vi "passIfReentrant.vi"(8 "error in (no error)":errorcluster, 9 "required setting (reentrant)":T1, 10 "VI Refnum":refnum<vi>, 11 "TestCase in":refnum<class "TestCase.lvclass">) -> (0 "error out":errorcluster, 3 "TestCase out":refnum<class "TestCase.lvclass">)   [LabVIEW 2013, in "EasyXML_XML_Subset_Evaluations.lvclass"]
doc: "Tests whether the VI specified by <b>VI Refnum</b> is reentrant or non-reentrant, as specified by <b>required setting</b>"
uses:
  EasyXML_XML_Subset_Evaluations.lvclass
  <vilib>/addons/_JKI Toolkits/VI Tester/TestCase.llb/TestCase.lvclass
  EasyXMLTest/Test Support/Reentrant Setting Requirement - Enum.ctl
  EasyXMLTest/EasyXMLTest.lvclass
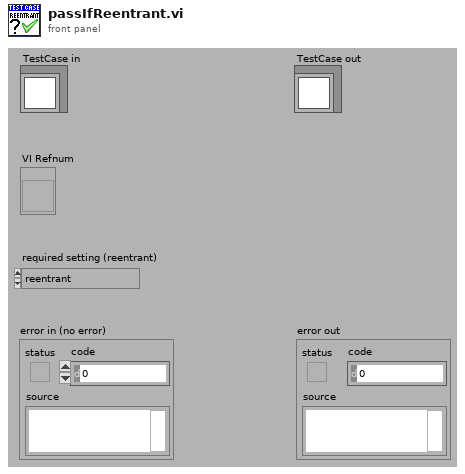
[diagram p1: front panel]
types:
  T1 = typedef "EasyXMLTest.lvclass/Reentrant Setting Requirement - Enum.ctl" = enum16{"reentrant", "non-reentrant"}
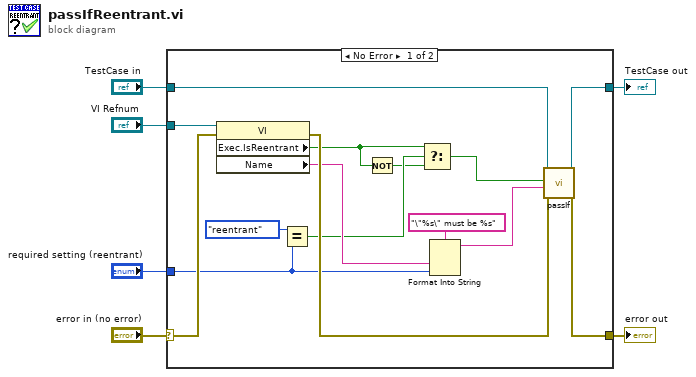
[diagram p0: block diagram]
diagram:
  n1 = case shown="No Error" "error in (no error)" {
    selector: "error in (no error)" -> [w13 w23]
    tunnel: [w19 w23] -> w5
    tunnel: [w18 w22] -> w4
    tunnel: "TestCase in" -> [w17 w22]
    tunnel: "VI Refnum" -> [w14 _]
    tunnel: "required setting (reentrant)" -> [w11 _]
    frame No Error {
      n2 = property class="VI"(reference=w14, error in=w13) -> (error out=w21:errorcluster, "Exec.IsReentrant"=w8:bool, "Name"=w15:string)  [unwired: 1 out]
      n3 = Equal?(x=Reentrant_Setting_Requirement_-_Enum."reentrant" ("required setting (reentrant)"), y=w11) -> (x = y?=w10:bool)
      n4 = Not(x=w8) -> (.not. x?=w7:bool)
      n5 = Select(t=w8, s=w10, f=w7) -> (s? t:f=w9:bool)
      n6 = Format Into String(format string="\"%s\" must be %s", w15, w11) -> (resulting string=w20:string)  [unwired: 2 in, 1 out]
      n7 = call-dynamic "passIf.vi"("error in (no error)"=w21, "message (\"\")"=w20, "pass"=w9, "TestCase in"=w17) -> ("error out"=w19:errorcluster, "TestCase out"=w18:refnum<class "TestCase.lvclass">)  [unwired: 6 in]
    }
    frame Error {
    }
  }
  "error out" <- w5
  "TestCase out" <- w4
